vi "shift_below_1_OLD.vi"(9 "input valid":bool, 10 "input":fxp<+/-,64,32>) -> (0 "ready for input":bool=TRUE, 1 "output valid":bool, 2 "shifted":fxp<+/-,64,32>, 3 "count":i16)   [LabVIEW 2018]
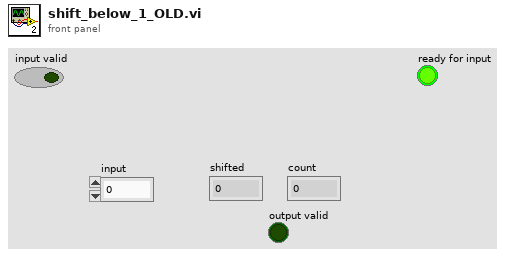
[diagram p1: front panel]
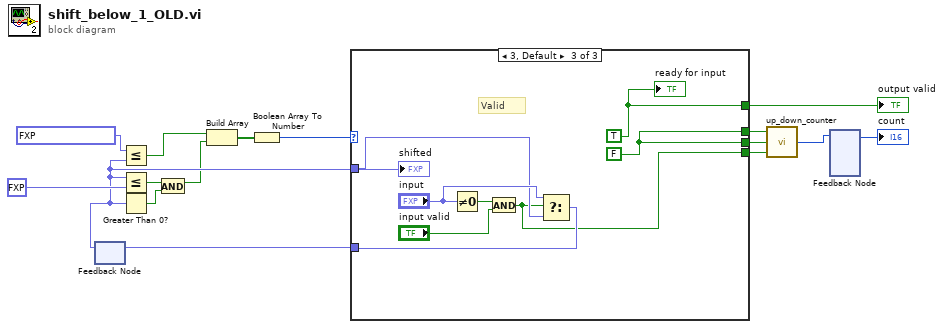
[diagram p0: block diagram]
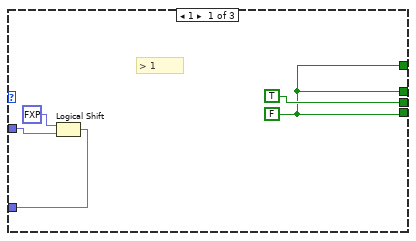
[diagram p2: hidden frame]
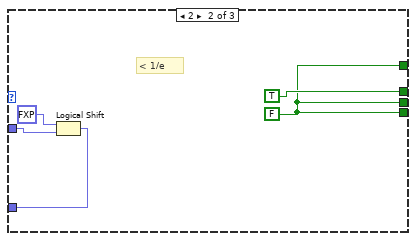
[diagram p3: hidden frame]
diagram:
  n1 = feedback #1() -> (w3:fxp<+/-,64,32>)  [unwired: 1 in]
  n2 = Less Or Equal?(x=fxp<+,16,-1> 0.36785888671875, y=w3) -> (x <= y?=w11:bool)
  n3 = Less Or Equal?(x=w3, y=fxp<+,1,1> 1.0) -> (x <= y?=w12:bool)
  n4 = Greater Than 0?(x=w3) -> (x > 0?=w1:bool)
  n5 = And(x=w12, y=w1) -> (x .and. y?=w2:bool)
  n6 = Build Array(w11, w2) -> (w13:bool[])
  n7 = Boolean Array To Number(Boolean array=w13) -> (number=w14:u8)
  n8 = case shown="3, Default" w14 {
    tunnel: w3 -> [w21 w26 w30]
    tunnel: [w18 w23 w27] -> w10
    tunnel: [TRUE w23 w34] -> w9
    tunnel: [w18 TRUE w34] -> w8
    tunnel: [w18 w23 w28] -> w5
    tunnel: [w17 w22 w29] -> w4
    frame 1 {
      w18 = FALSE
      # "> 1"
      n9 = Logical Shift(y=fxp<+/-,1,1> -1.0, x=w21) -> (x << y=w17:fxp<+/-,64,32>)
    }
    frame 2 {
      w23 = FALSE
      # "< 1/e"
      n10 = Logical Shift(y=fxp<+,1,1> 1.0, x=w26) -> (x << y=w22:fxp<+/-,64,32>)
    }
    frame 3, Default {
      w34 = FALSE
      w28 = TRUE
      # "Valid"
      n11 = Not Equal To 0?(x="input") -> (x != 0?=w33:bool)
      n12 = And(x=w33, y="input valid") -> (x .and. y?=w27:bool)
      n13 = Select(t="input", s=w27, f=w30) -> (s? t:f=w29:fxp<+/-,64,32>)
      "shifted" <- w30
      "ready for input" <- w28
    }
  }
  "output valid" <- w5
  n14 = feedback-in #1(w4) -> ()
  n15 = call "up_down_counter.vi"("reset"=w10, "up"=w9, "down"=w8) -> ("Value"=w7:i16)
  n16 = feedback #2() -> (→"count":i16)  [unwired: 1 in]
  n17 = feedback-in #2(w7) -> ()
